vi "main.vi"() -> ()   [LabVIEW 2023]
uses:
  #typedef_state.ctl
  <vilib>/event_ctls.llb/lveventtype.ctl
  #typedef_data.ctl
  <vilib>/Utility/miscctls.llb/LVPositionTypeDef.ctl
panel:
  out "current code [max 4]":string
  out "Limit exceeded ?":bool
  in  "Sound intensity: MAX":dbl
  in  "Sound intensity: MIN":dbl
  in  "Sound Intensity [dB]":dbl(slide) min=40.0 max=100.0 scale=20.0..100.0
  in  "Stop Button":bool
  out "Play Button":bool
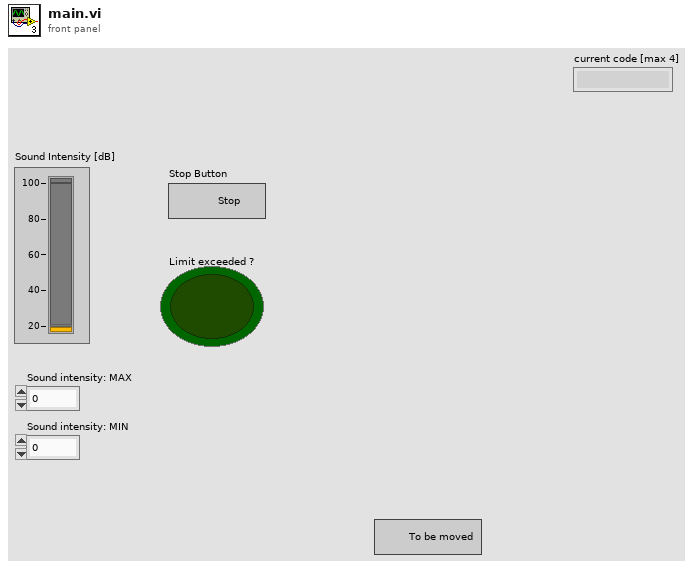
[diagram p1: front panel]
types:
  T1 = typedef "#typedef_state.ctl" = enum16{"Aplication error", "Change ", "Idling", "Intensity check", "Inicializing", "Exit"}
  T2 = typedef "lveventtype.ctl" = enum32{"Null", "Timeout", "Annotation Menu Selection", "Annotation Menu Selection?", "App Instance Close", "App Instance Close?", "Autoscale Range Change", "Bookmark Info Change", "Cell Edit", "Cell Edit?", "Cursor Grab", "Cursor Grab?", "Cursor Menu Selection", "Cursor Menu Selection?", "Cursor Move", "Cursor Release", "Data Change", "Direction Change", "Display State Change", "Drag Ended", "Drag Enter", "Drag Leave", "Drag Over", "Drag Source Update", "Drag Starting", "Drag Starting?", "Drop", "Exec State Change", "Key Down", "Key Down?", "Key Repeat", "Key Repeat?", "Key Up", "Listbox Double Click", "Menu Activation?", "Menu Selection (App)", "Menu Selection? (App)", "Menu Selection (User)", "Mouse Down", "Mouse Down?", "Mouse Enter", "Mouse Leave", "Mouse Move", "Mouse Up", "Mouse Wheel", "NI Security User Change (App)", "Pane Size", "Panel Close", "Panel Close?", "Panel Resize", "Plot Attribute Change", "Scale Range Change", "Shortcut Menu Activation?", "Shortcut Menu Selection (App)", "Shortcut Menu Selection? (App)", "Shortcut Menu Selection (User)", "Tree Double Click", "Tree Drag", "Tree Drag?", "Tree Drop", "Tree Drop?", "Tree Item Close", "Tree Item Close?", "Tree Item Open", "Tree Item Open?", "User Event", "Value Change"}
  T3 = typedef "#typedef_data.ctl" = cluster{"Sound Intensity [dB]":dbl, "Sound intensity: MIN":dbl, "Sound intensity: MAX":dbl, "Limit exceeded ?":bool, "MovingNow":bool, "PositionOfset":T4, "Position ":T4, "Kod":string}
  T4 = typedef "LVPositionTypeDef.ctl" = cluster{"Left":i32, "Top":i32}
  T5 = typedef "LVPoint32TypeDef.ctl" = cluster{"Horizontal":i32, "Vertical":i32}
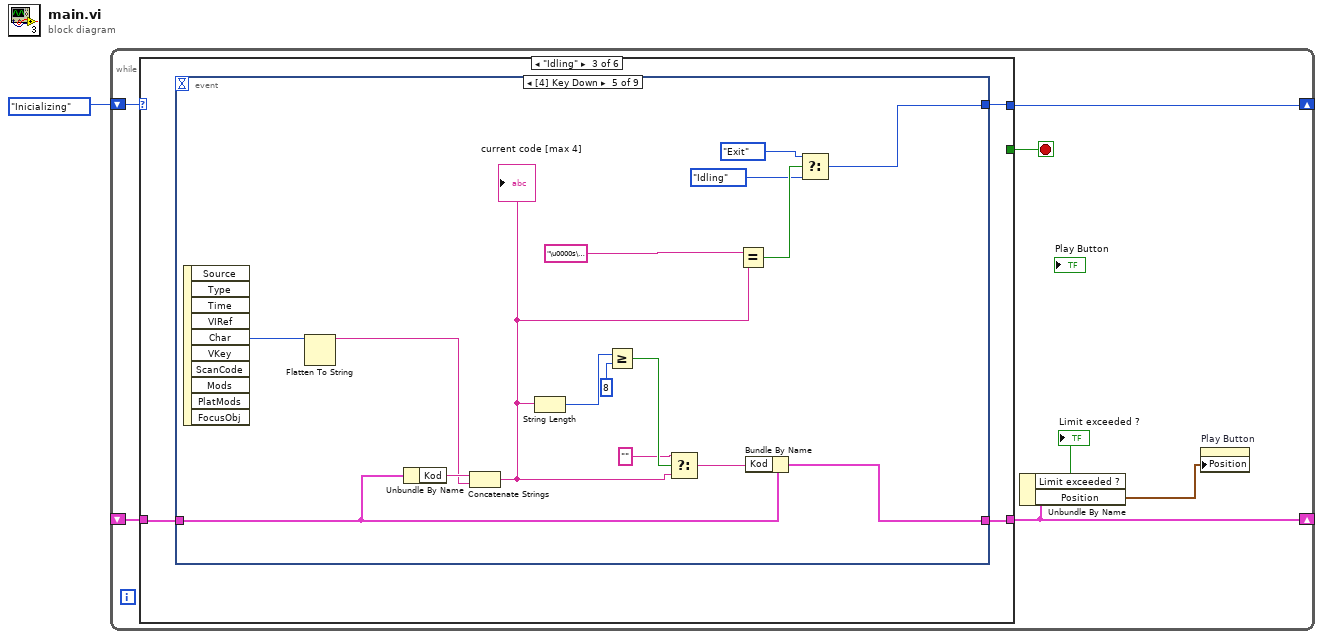
[diagram p0: block diagram]
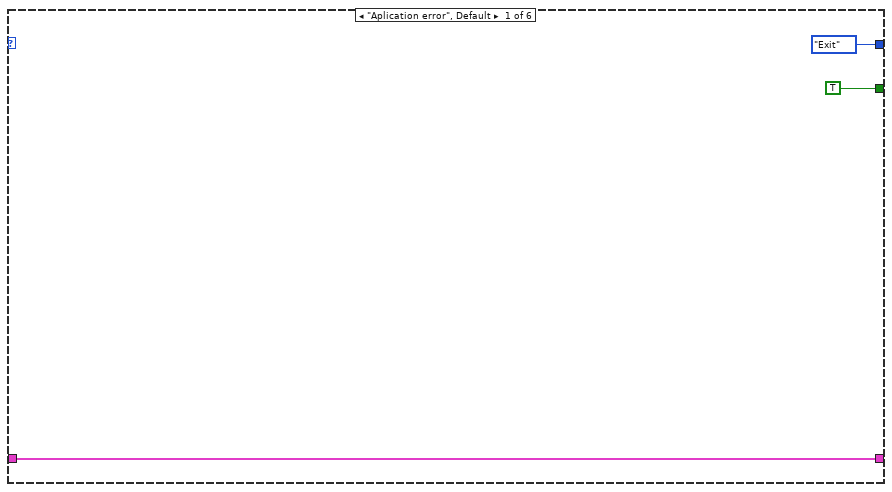
[diagram p2: hidden frame]
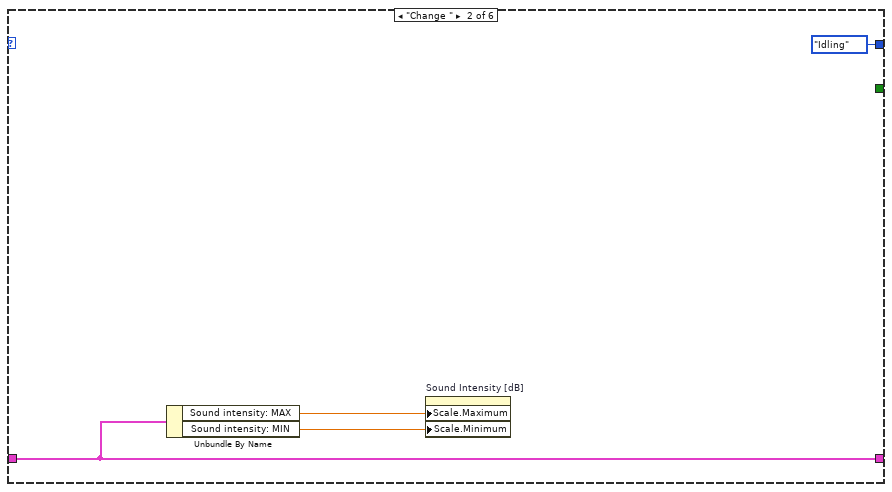
[diagram p3: hidden frame]
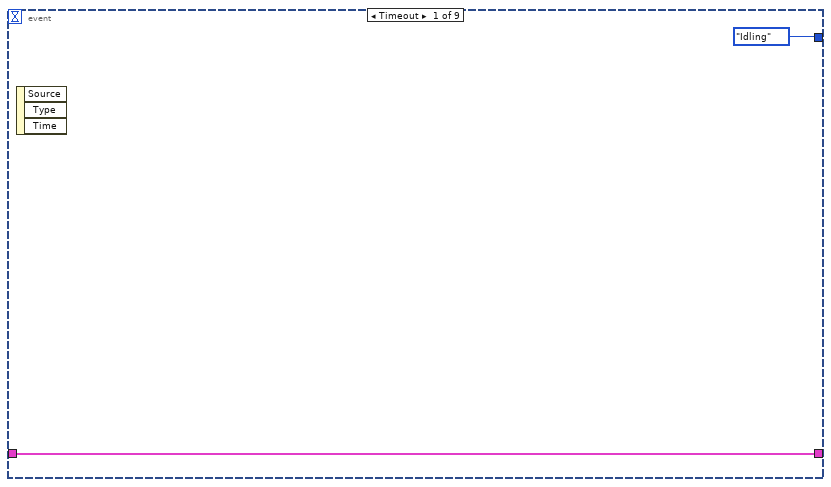
[diagram p4: hidden frame]
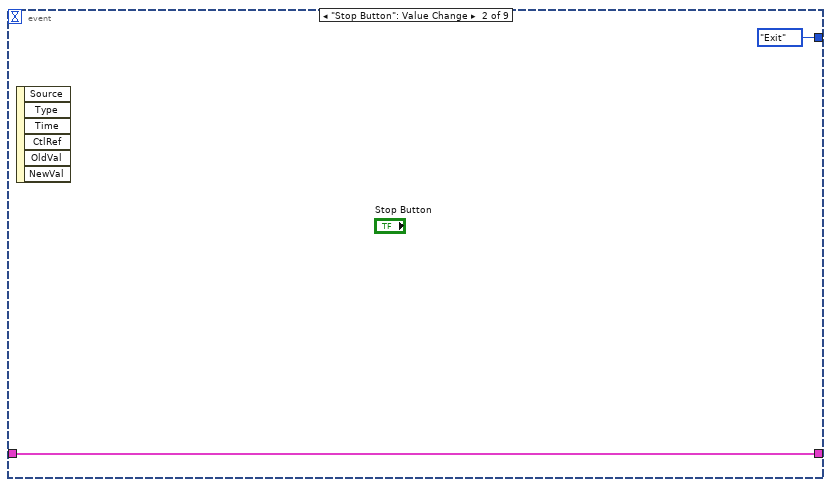
[diagram p5: hidden frame]
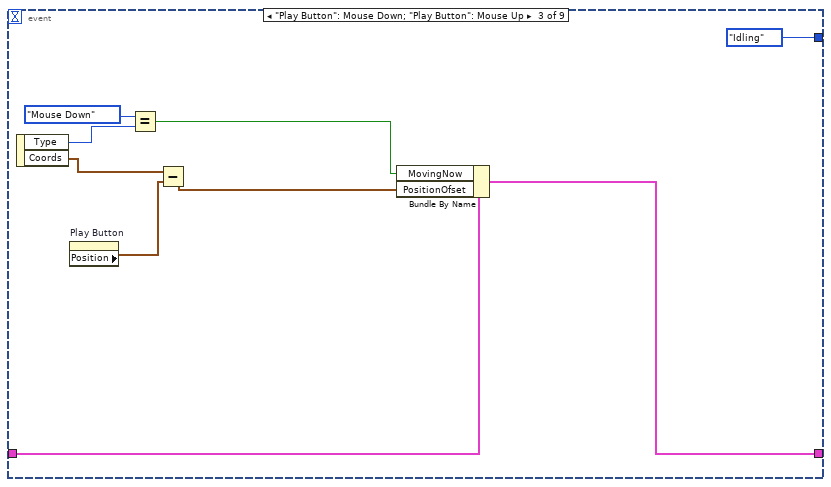
[diagram p6: hidden frame]
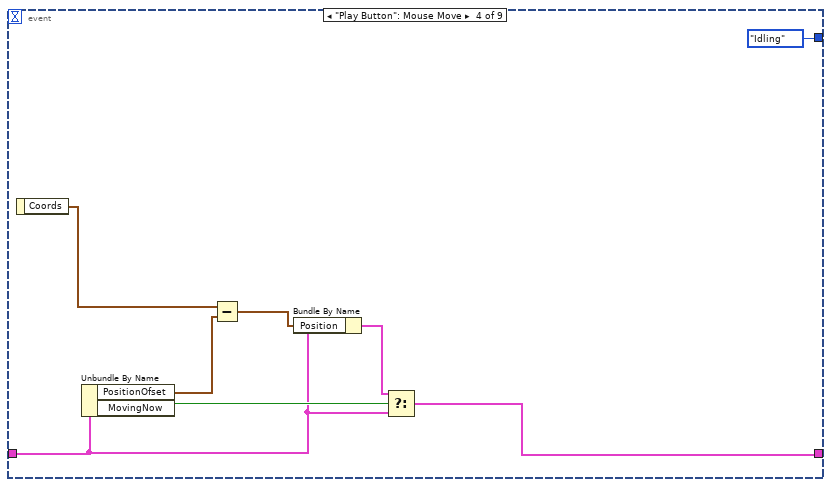
[diagram p7: hidden frame]
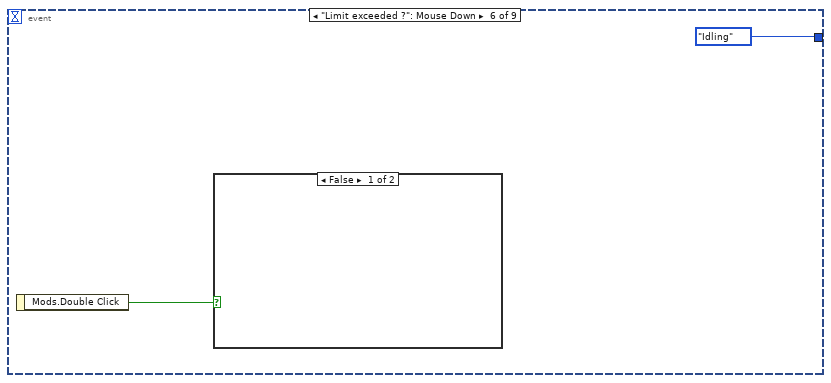
[diagram p8: hidden frame]
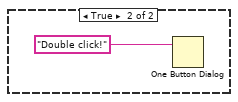
[diagram p9: hidden frame]
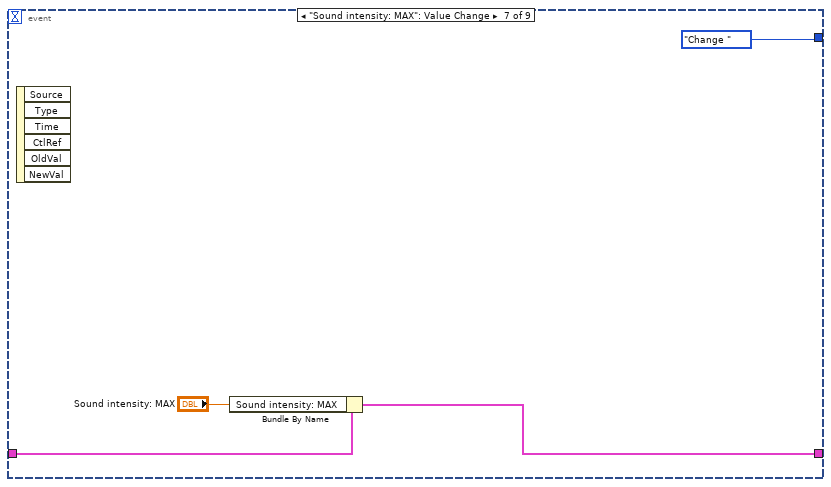
[diagram p10: hidden frame]
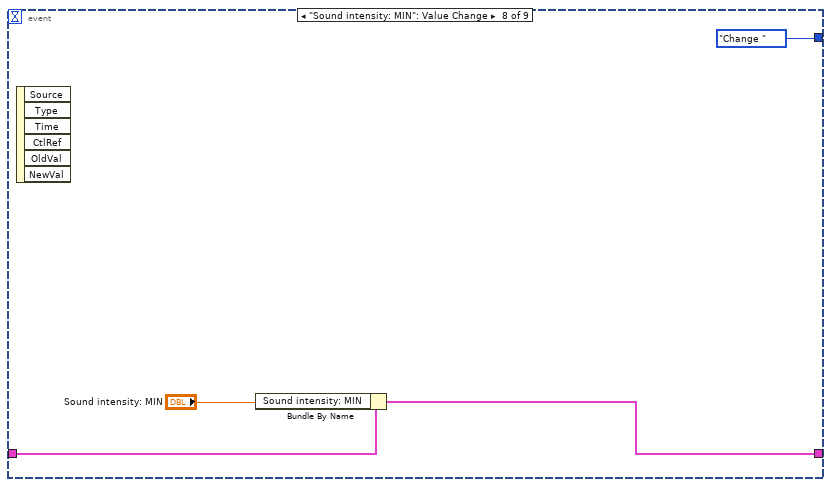
[diagram p11: hidden frame]
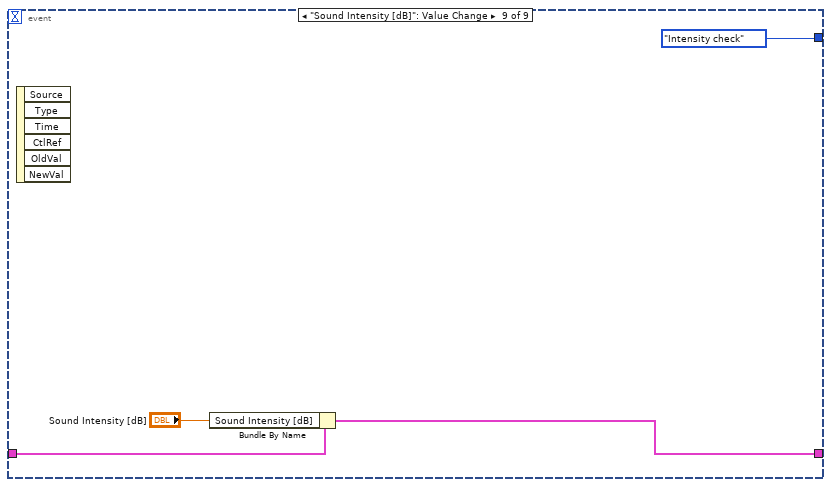
[diagram p12: hidden frame]
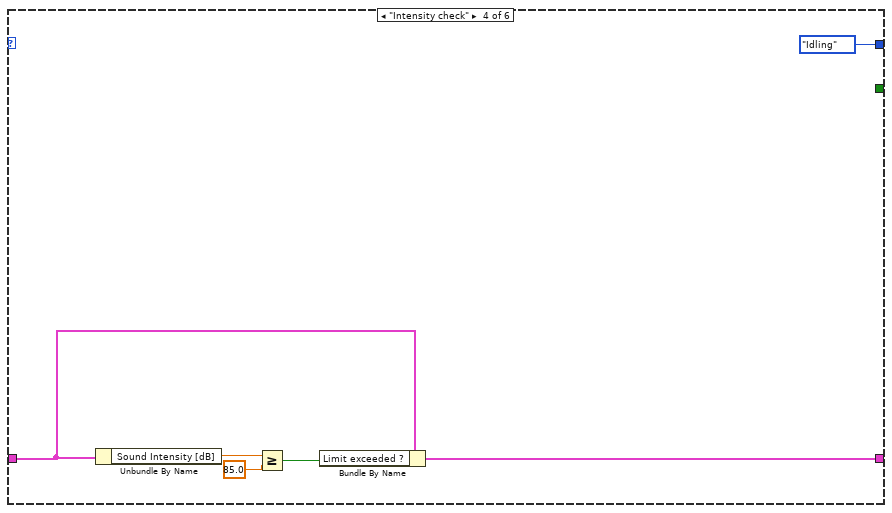
[diagram p13: hidden frame]
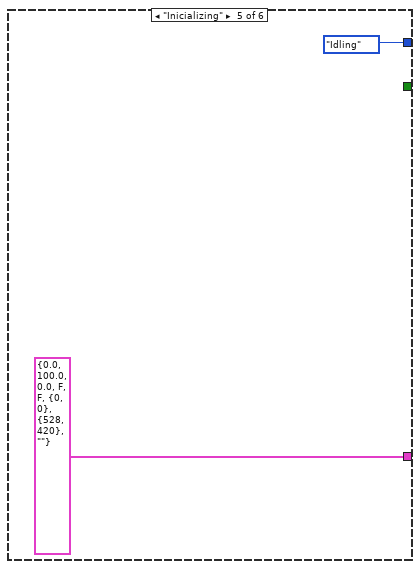
[diagram p14: hidden frame]
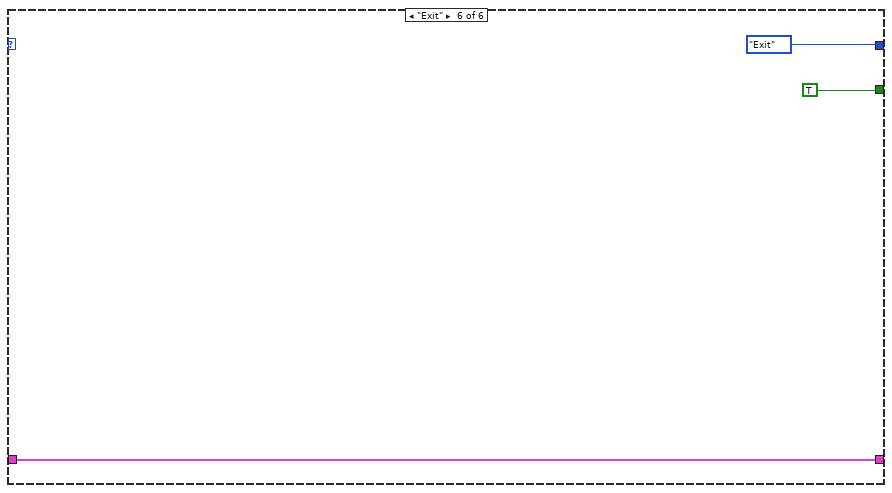
[diagram p15: hidden frame]
diagram:
  n1 = while {
    shift-right: [w7] -> _
    shift-left: #typedef_state."Inicializing" ("State") -> [w8]
    shift-right: [w4] -> _
    shift-left: _ -> [w6]
    stop <- w5 stop-if-true
    n2 = case shown="\"Idling\"" w8 {
      tunnel: [#typedef_state."Exit" ("State") #typedef_state."Idling" ("State") w18 #typedef_state."Idling" ("State") #typedef_state."Idling" ("State") #typedef_state."Exit" ("State")] -> w7
      tunnel: [w10 w14 w16 w72 T3 {"Sound Intensity [dB]"=0.0, "Sound intensity: MIN"=100.0, "Sound intensity: MAX"=0.0, "Limit exceeded ?"=FALSE, "MovingNow"=FALSE, "PositionOfset"={"Left"=0, "Top"=0}, "Position "={"Left"=528, "Top"=420}, "Kod"=""} ("Data") w81] -> w4
      tunnel: w6 -> [w10 w14 w17 w73 _ w81]
      tunnel: [TRUE _ _ _ _ TRUE] -> w5
      frame "Aplication error", Default {
      }
      frame "Change " {
        n3 = Unbundle By Name(w14) -> ("Sound intensity: MAX"=w13:dbl, "Sound intensity: MIN"=w12:dbl)
        n4 = property on="Sound Intensity [dB]" class="Slide (strict)"("Scale.Maximum"=w13, "Scale.Minimum"=w12) -> ()  [unwired: 2 in, 2 out]
      }
      frame "Idling" {
        n5 = event shown="[4] Key Down" {
          selector: _ -> [_ _ _ _ _ _ _ _ _]
          dyn-events: _ -> [_ _ _ _ _ _ _ _ _]
          timeout: _ -> [_ _ _ _ _ _ _ _ _]
          tunnel: [#typedef_state."Idling" ("State") #typedef_state."Exit" ("State") #typedef_state."Idling" ("State") #typedef_state."Idling" ("State") w42 #typedef_state."Idling" ("State") #typedef_state."Change " ("State") #typedef_state."Change " ("State") #typedef_state."Intensity check" ("State")] -> w18
          tunnel: w17 -> [w19 w21 w27 w37 w48 _ w62 w66 w69]
          tunnel: [w19 w21 w26 w38 w47 _ w60 w64 w67] -> w16
          event Timeout {
            n6 = event-data() -> ()  [unwired: 1 in, 3 out]
          }
          event "Stop Button": Value Change {
            n7 = event-data() -> ()  [unwired: 1 in, 6 out]
          }
          event "Play Button": Mouse Down; "Play Button": Mouse Up {
            n8 = event-data() -> ("Type"=w31:T2, "Coords"=w29:T5)  [unwired: 1 in]
            n9 = property on="Play Button" class="Bool"() -> ("Position"=w28:T4)  [unwired: 2 in, 2 out]
            n10 = Equal?(x=lveventtype."Mouse Down", y=w31) -> (x = y?=w24:bool)
            n11 = Subtract(x=w29, y=w28) -> (x-y=w25:T5)
            n12 = Bundle By Name(cluster=w27, "MovingNow"=w24, "PositionOfset"=w25) -> (w26:T3)
          }
          event "Play Button": Mouse Move {
            n13 = event-data() -> ("Coords"=w34:T5)  [unwired: 1 in]
            n14 = Unbundle By Name(w37) -> ("PositionOfset"=w33:T4, "MovingNow"=w39:bool)
            n15 = Subtract(x=w34, y=w33) -> (x-y=w32:T5)
            n16 = Bundle By Name(cluster=w37, "Position"=w32) -> (w36:T3)
            n17 = Select(t=w36, s=w39, f=w37) -> (s? t:f=w38:T3)
          }
          event Key Down {
            n18 = event-data() -> ("Char"=w55:i16)  [unwired: 1 in, 9 out]
            n19 = Flatten To String(anything=w55) -> (data string=w53:string)  [unwired: 3 in, 2 out]
            n20 = Unbundle By Name(w48) -> ("Kod"=w54:string)
            n21 = Concatenate Strings(w54, w53) -> (w40:string)
            "current code [max 4]" <- w40
            n22 = String Length(string=w40) -> (length=w52:i32)
            n23 = Greater Or Equal?(x=w52, y=8) -> (x >= y?=w50:bool)
            n24 = Select(t="", s=w50, f=w40) -> (s? t:f=w41:string)
            n25 = Equal?(x="\u0000s\u0000t\u0000o\u0000p", y=w40) -> (x = y?=w45:bool)
            n26 = Bundle By Name(cluster=w48, "Kod"=w41) -> (w47:T3)
            n27 = Select(t=#typedef_state."Exit", s=w45, f=#typedef_state."Idling" ("State")) -> (s? t:f=w42:T1)
          }
          event "Limit exceeded ?": Mouse Down {
            n28 = event-data() -> ("Mods.Double Click"=w56:bool)  [unwired: 1 in]
            n29 = case shown="False" w56 {
              frame False {
              }
              frame True {
                n30 = One Button Dialog(message="Double click!") -> ()  [unwired: 1 in, 1 out]
              }
            }
          }
          event "Sound intensity: MAX": Value Change {
            n31 = event-data() -> ()  [unwired: 1 in, 6 out]
            n32 = Bundle By Name(cluster=w62, "Sound intensity: MAX"="Sound intensity: MAX") -> (w60:T3)
          }
          event "Sound intensity: MIN": Value Change {
            n33 = event-data() -> ()  [unwired: 1 in, 6 out]
            n34 = Bundle By Name(cluster=w66, "Sound intensity: MIN"="Sound intensity: MIN") -> (w64:T3)
          }
          event "Sound Intensity [dB]": Value Change {
            n35 = event-data() -> ()  [unwired: 1 in, 6 out]
            n36 = Bundle By Name(cluster=w69, "Sound Intensity [dB]"="Sound Intensity [dB]") -> (w67:T3)
          }
        }
      }
      frame "Intensity check" {
        n37 = Unbundle By Name(w73) -> ("Sound Intensity [dB]"=w76:dbl)
        n38 = Greater Or Equal?(x=w76, y=85.0) -> (x >= y?=w74:bool)
        n39 = Bundle By Name(cluster=w73, "Limit exceeded ?"=w74) -> (w72:T3)
      }
      frame "Inicializing" {
      }
      frame "Exit" {
      }
    }
    n40 = Unbundle By Name(w4) -> ("Limit exceeded ?"=→"Limit exceeded ?":bool, "Position"=w2:T4)
    n41 = property on="Play Button" class="Bool"("Position"=w2) -> ()  [unwired: 2 in, 2 out]
  }
